vi "Downconvert.vi"(8 "error in (no error)":errorcluster, 9 "passband bandwidth (Hz)":dbl format="%.2p", 10 "carrier frequency (Hz)":dbl min=-0.5 max=0.5 format="%.2p", 11 "CDB Wfm in":waveform(cdb)) -> (0 "error out":errorcluster, 3 "CDB Wfm out":waveform(cdb))   [LabVIEW 2015, in "Monitoring_receiver.lvlib"]
uses:
  <vilib>/addons/Modulation/Analog/controls/Complex Data Waveform.ctl
  <vilib>/addons/Modulation/Analog/support/Validators/mod_Fractional Resample Validate.vi
  <vilib>/addons/Modulation/Analog/support/Validators/mod_Check Flush State.vi
  <vilib>/addons/Modulation/Analog/support/mod_FractionalResampler.vi
  <vilib>/addons/Modulation/Analog/support/mod_Integer Rate Interpolation.vi
  <vilib>/addons/Modulation/Analog/support/mod_Set Error Source.vi
  <vilib>/addons/Modulation/Analog/support/Validators/mod_Validate Complex Waveform.vi
  <vilib>/addons/Modulation/Analog/support/mod_PerformResampling.vi
  <vilib>/addons/Modulation/Analog/support/Validators/mod_WFErrorHandler.vi
  <vilib>/addons/Modulation/Analog/MT Downconvert Passband (Complex).vi
  <vilib>/Analysis/2dsp.llb/Decimate (continuous, DBL).vi
  <vilib>/Utility/error.llb/Error Cluster From Error Code.vi
  <vilib>/addons/Modulation/Analog/support/mod_Resampling Factors.vi
  <vilib>/addons/Modulation/Analog/support/mod_ResamplingFilter.vi
  <vilib>/addons/Modulation/Analog/support/mod_Generate Integer Interpolation Filter.vi
  Monitoring_receiver.lvlib
  <vilib>/addons/Modulation/niAMT.lvlib
  <vilib>/Analysis/NI_AALPro.lvlib
panel:
  out "Sample rate out":dbl
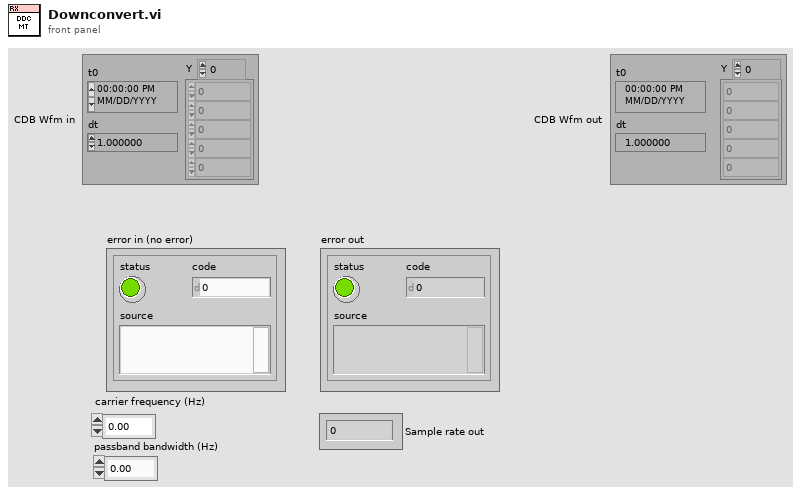
[diagram p1: front panel]
types:
  T1 = cluster{"passband ripple (dB)":dbl, "stopband start (Hz)":dbl, "stopband gain (dB)":dbl, "compute filter stopband ? (T)":bool}
  T2 = typedef "niAMT.lvlib/Complex Data Waveform.ctl" = cluster{"t0":dbl, "dt":dbl, "Y":cdb[]}
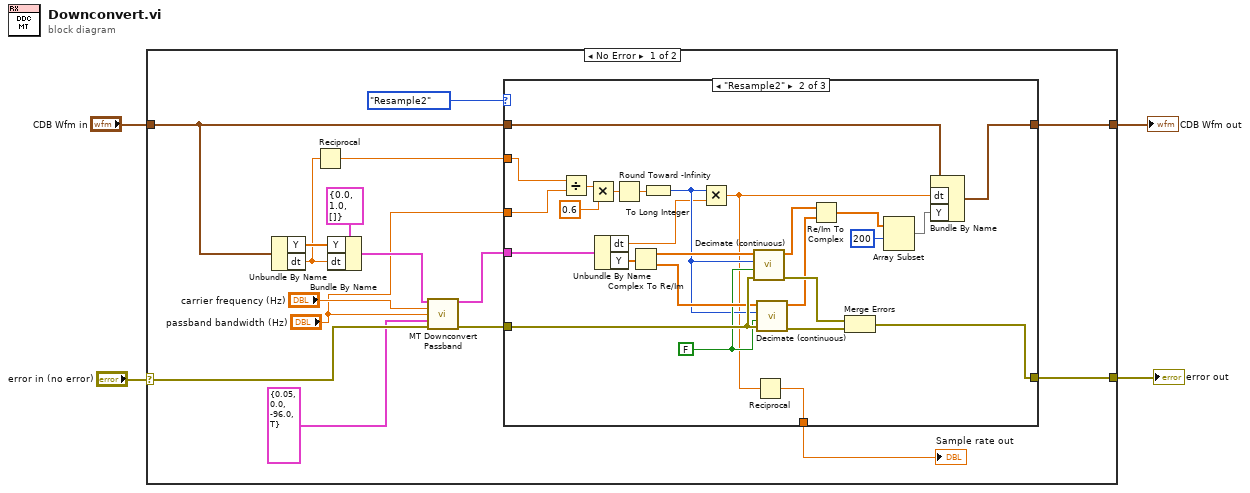
[diagram p0: block diagram]
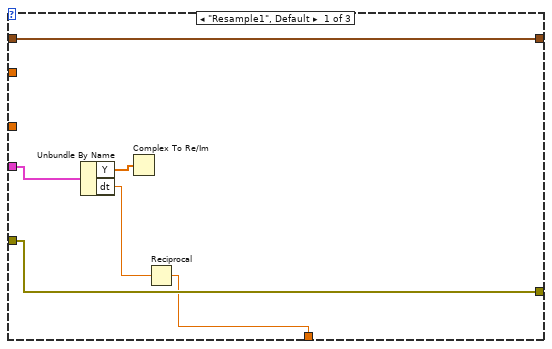
[diagram p2: hidden frame]
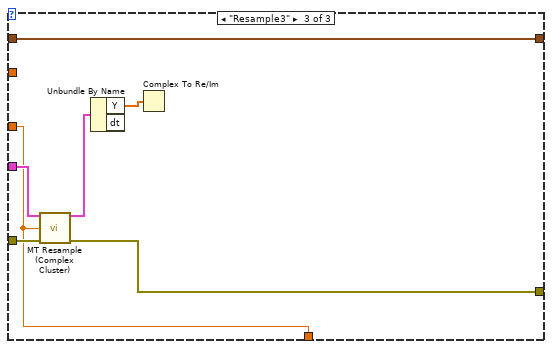
[diagram p3: hidden frame]
diagram:
  n1 = case shown="No Error" "error in (no error)" {
    selector: "error in (no error)" -> [w18 w61]
    tunnel: [w15 w61] -> w4
    tunnel: "CDB Wfm in" -> [w6 w60]
    tunnel: [w5 w60] -> w1
    frame No Error {
      n2 = Unbundle By Name(w6) -> ("Y"=w9:cdb[], "dt"=w8:dbl)
      n3 = Reciprocal(x=w8) -> (1/x=w7:dbl)
      n4 = Bundle By Name(cluster=T2 {"t0"=0.0, "dt"=1.0, "Y"=[]} ("complex waveform"), "Y"=w9, "dt"=w8) -> (w19:T2)
      n5 = call-poly <vilib>:"MT Downconvert Passband.vi"("complex waveform"=w19, "carrier frequency (Hz)"="carrier frequency (Hz)", "passband bandwidth (Hz)"="passband bandwidth (Hz)", "advanced filter parameters"=T1 {"passband ripple (dB)"=0.05, "stopband start (Hz)"=0.0, "stopband gain (dB)"=-96.0, "compute filter stopband ? (T)"=TRUE}, "error in (no error)"=w18) -> ("downconverted waveform (complex)"=w14:T2, "error out"=w16:errorcluster)  [unwired: 7 in, 2 out]
      n6 = case shown="\"Resample2\"" enum16{"Resample1", "Resample2", "Resample3"}."Resample2" {
        tunnel: w16 -> [w26 w52 w56]
        tunnel: [w26 w36 w55] -> w15
        tunnel: w14 -> [w24 w51 w57]
        tunnel: [w22 w44 w54] -> w10
        tunnel: "passband bandwidth (Hz)" -> [_ w42 w54]
        tunnel: w7 -> [_ w43 _]
        tunnel: w6 -> [w21 w32 w53]
        tunnel: [w21 w31 w53] -> w5
        frame "Resample1", Default {
          n7 = Unbundle By Name(w24) -> ("Y"=w25:cdb[], "dt"=w23:dbl)
          n8 = Complex To Re/Im(x + iy=w25) -> ()  [unwired: 2 out]
          n9 = Reciprocal(x=w23) -> (1/x=w22:dbl)
        }
        frame "Resample2" {
          w47 = FALSE ("averaging")
          n10 = Divide(x=w43, y=w42) -> (x/y=w41:dbl)
          n11 = Multiply(x=w41, y=0.6) -> (x*y=w39:dbl)
          n12 = Unbundle By Name(w51) -> ("dt"=w30:dbl, "Y"=w50:cdb[])
          n13 = Round Toward -Infinity(1:w39) -> (0:w38:dbl)
          n14 = Complex To Re/Im(x + iy=w50) -> (x=w49:dbl[], y=w48:dbl[])
          n15 = To Long Integer(number=w38) -> (32bit integer=w37:i32)
          n16 = Multiply(x=w37, y=w30) -> (x*y=w33:dbl)
          n17 = call-poly <vilib>:"Decimate (continuous).vi"("error in (no error)"=w52, "averaging"=w47, "decimating factor"=w37, "X"=w49) -> ("error out"=w46:errorcluster, "Decimated Array"=w35:dbl[])  [unwired: 6 in]
          n18 = Reciprocal(x=w33) -> (1/x=w44:dbl)
          n19 = call-poly <vilib>:"Decimate (continuous).vi"("error in (no error)"=w52, "averaging"=w47, "decimating factor"=w37, "X"=w48) -> ("error out"=w45:errorcluster, "Decimated Array"=w34:dbl[])  [unwired: 6 in]
          n20 = Re/Im To Complex(1:w34, 2:w35) -> (0:w29:cdb[])
          n21 = Merge Errors(w46, w45) -> (w36:errorcluster)
          n22 = Array Subset(array=w29, index=200) -> (w27:cdb[])  [unwired: 1 in]
          n23 = Bundle By Name(cluster=w32, "dt"=w33, "Y"=w27) -> (w31:waveform(cdb))
        }
        frame "Resample3" {
          n24 = call <vilib>:"MT Resample (Complex Cluster).vi"("input complex waveform"=w57, "desired sample rate (Hz)"=w54, "error in (no error)"=w56) -> ("output complex waveform"=w58:T2, "error out"=w55:errorcluster)  [unwired: 11 in]
          n25 = Unbundle By Name(w58) -> ("Y"=w59:cdb[])  [unwired: 1 out]
          n26 = Complex To Re/Im(x + iy=w59) -> ()  [unwired: 2 out]
        }
      }
      "Sample rate out" <- w10
    }
    frame Error {
    }
  }
  "error out" <- w4
  "CDB Wfm out" <- w1
